vi "Read Subscriptions.vi"(11 "MVC Subscription in":refnum<class "MVC Subscription.lvclass">) -> (2 "Subscriptions":T1[](array[typedef]), 3 "MVC Subscription out":refnum<class "MVC Subscription.lvclass">)   [LabVIEW 2014, in "MVC Subscription.lvlib" / "MVC Subscription.lvclass"]
uses:
  MVC Subscription.lvclass
  Cluster - Individual Subscription.ctl
  <vilib>/ActorFramework/Message Enqueuer/Message Enqueuer.lvclass
  <vilib>/ActorFramework/Message/Message.lvclass
  MVC Subscription.lvclass/MVC Subscription.ctl
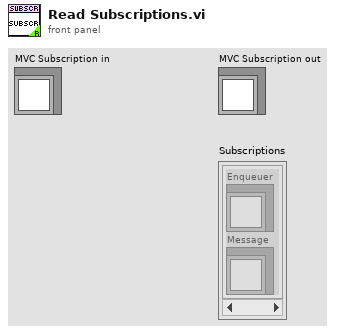
[diagram p1: front panel]
types:
  T1 = typedef "MVC Subscription.lvlib/MVC Subscription.lvclass/Cluster - Individual Subscription.ctl" = cluster{"Enqueuer":refnum<class "Message Enqueuer.lvclass">, "Message":refnum<class "Message.lvclass">}
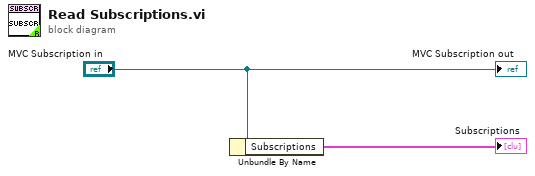
[diagram p0: block diagram]
diagram:
  n1 = Unbundle By Name("MVC Subscription in") -> ("Subscriptions"=→"Subscriptions":T1[])
  "MVC Subscription out" <- "MVC Subscription in"
